vi "Continuous B-Scan Demo.vi"() -> ()   [LabVIEW 2012]
uses:
  LabVIEW/user.lib/SpectralRadar.llb/Device Camera Preset Selection.ctl
  LabVIEW/user.lib/SpectralRadar.llb/Raw Data Export Format Selection.ctl
  LabVIEW/user.lib/SpectralRadar.llb/set Spectrum Output.vi
  LabVIEW/user.lib/SpectralRadar.llb/set Scan Output.vi
  LabVIEW/user.lib/SpectralRadar.llb/display Data 2D.vi
  LabVIEW/user.lib/SpectralRadar.llb/OCT Device.lvclass
  LabVIEW/user.lib/SpectralRadar.llb/Probe.lvclass
  LabVIEW/user.lib/SpectralRadar.llb/Processing.lvclass
  LabVIEW/user.lib/SpectralRadar.llb/Raw Data.lvclass
  LabVIEW/user.lib/SpectralRadar.llb/Data.lvclass
  LabVIEW/user.lib/SpectralRadar.llb/Scan Pattern.lvclass
panel:
  in  "Raw Data Export Format":T1
  in  "Device Camera Preset":T2=enum."Preset 1"
  in  "Range":dbl=1.0
  in  "Path":path
  in  "stop":bool
  out "B-Scan Data":dbl[][](graph)
  out "Spectral Data":dbl[][](graph)
  in  "AScans":i32=512
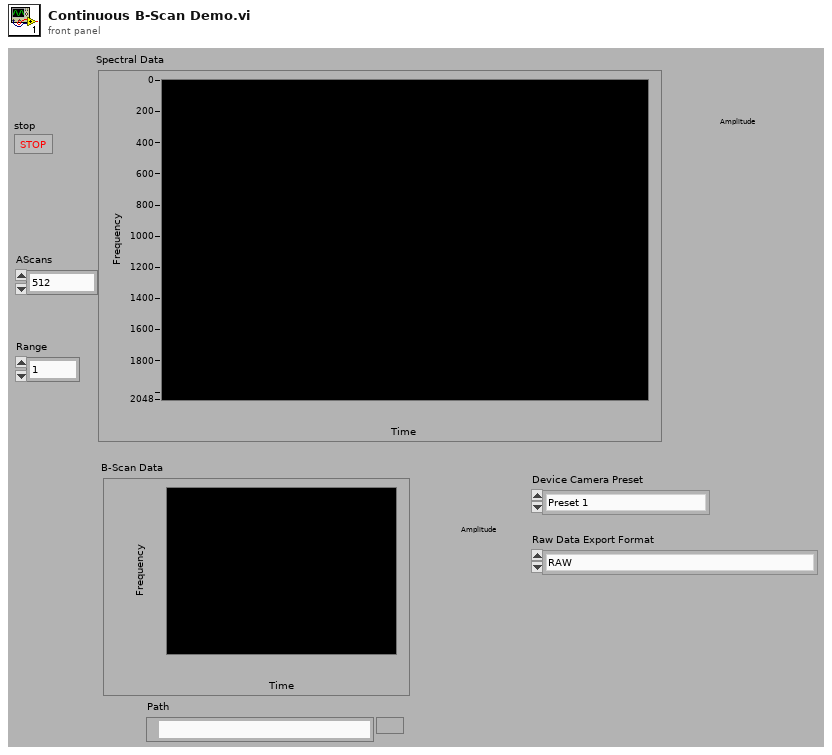
[diagram p1: front panel]
types:
  T1 = typedef "Raw Data.lvclass/Raw Data Export Format Selection.ctl" = enum16{"RAW", "SRR (Spectral Radar Raw)"}
  T2 = typedef "OCT Device.lvclass/Device Camera Preset Selection.ctl" = enum16{"Default", "Preset 1", "Preset 2", "Preset 3"}
  T3 = enum16{"Asynchronous Continuous", "Asynchronous Finite", "Synchronous"}
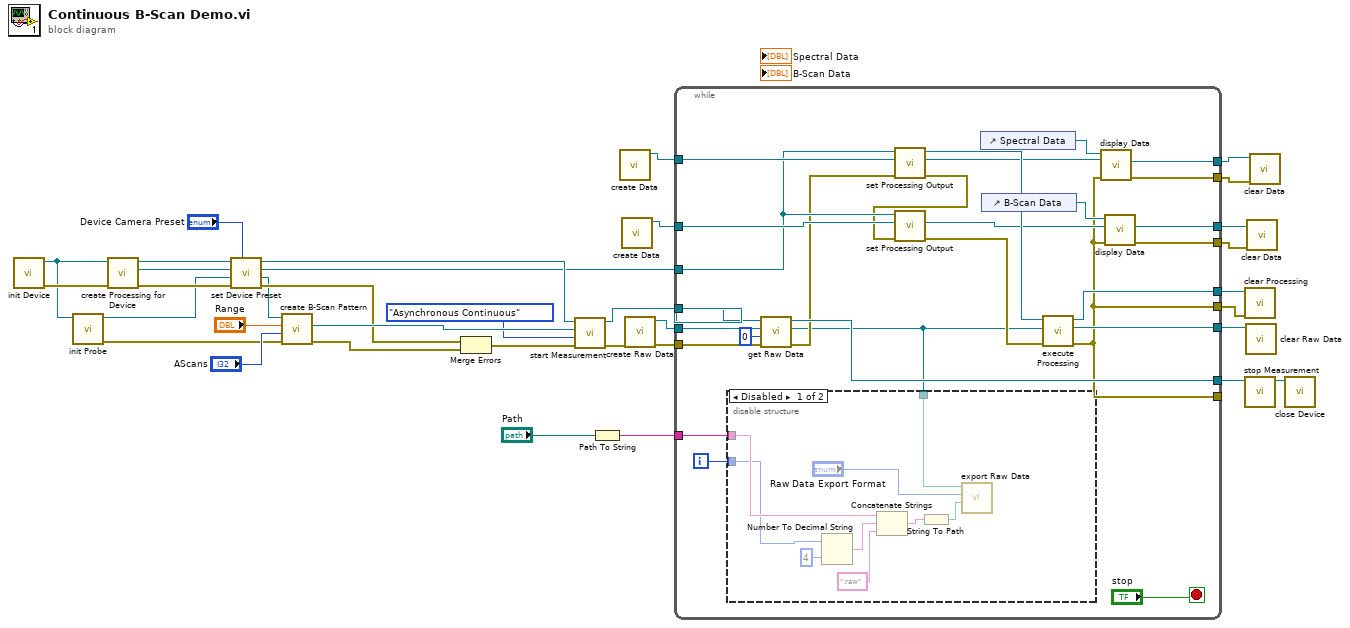
[diagram p0: block diagram]
diagram:
  n1 = call "init Device.vi"() -> ("error out"=w34:errorcluster, "OCTDevice"=w21:refnum<class "OCT Device.lvclass">)  [unwired: 6 in]
  n2 = call "init Probe.vi"("OCT Device"=w21) -> ("error out"=w20:errorcluster, "GalvoControl"=w15:refnum<class "Probe.lvclass">)  [unwired: 5 in]
  n3 = call "create Processing for Device.vi"("error in (no error)"=w34, "OCTDevice"=w21) -> ("error out"=w28:errorcluster, "Processing"=w13:refnum<class "Processing.lvclass">, "OCTDevice"=w16:refnum<class "OCT Device.lvclass">)  [unwired: 3 in]
  n4 = call "set Device Preset.vi"("Numeric"="Device Camera Preset", "Probe"=w15, "Processing"=w13, "OCTDevice"=w16) -> ("Probe 2"=w11:refnum<class "Probe.lvclass">, "Processing"=w12:refnum<class "Processing.lvclass">, "OCTDevice out"=w14:refnum<class "OCT Device.lvclass">)  [unwired: 2 in, 1 out]
  n5 = call "create B-Scan Pattern.vi"("error in (no error)"=w20, "AScans"="AScans", "Range"="Range", "Probe"=w11) -> ("error out"=w30:errorcluster, "Scan Pattern"=w32:refnum<class "Scan Pattern.lvclass">)  [unwired: 2 in, 1 out]
  n6 = Merge Errors(w28, w30) -> (w29:errorcluster)
  n7 = call "start Measurement.vi"("error in (no error)"=w29, "Acquisition Type"=T3."Asynchronous Continuous", "Scan Pattern"=w32, "OCTDevice"=w14) -> ("error out"=w26:errorcluster, "OCTDevice"=w17:refnum<class "OCT Device.lvclass">)  [unwired: 1 in, 1 out]
  n8 = Path To String(path="Path") -> (string=w9:string)
  n9 = call "create Data.vi"() -> ("Data"=w2:refnum<class "Data.lvclass">)  [unwired: 6 in, 1 out]
  n10 = call "create Data.vi"() -> ("Data"=w1:refnum<class "Data.lvclass">)  [unwired: 6 in, 1 out]
  n11 = call "create Raw Data.vi"("error in (no error)"=w26) -> ("error out"=w25:errorcluster, "Raw Data"=w27:refnum<class "Raw Data.lvclass">)  [unwired: 5 in]
  n12 = while {
    tunnel: w27 -> [w60]
    tunnel: w17 -> [w61]
    tunnel: w25 -> [w59]
    tunnel: w12 -> [w56]
    tunnel: w1 -> [w58]
    tunnel: w2 -> [w57]
    tunnel: [w48] -> w24
    tunnel: [w47] -> w23
    tunnel: [w46] -> w6
    tunnel: [w45] -> w4
    tunnel: [w44] -> w5
    tunnel: [w43] -> w3
    tunnel: [w42] -> w19
    tunnel: [w40] -> w22
    tunnel: [w40] -> _
    tunnel: w9 -> [w37]
    i -> [w36]
    stop <- "stop" stop-if-true
    n13 = call "get Raw Data.vi"("error in (no error)"=w59, "Camera Index"=0, "RawData in"=w60, "OCTDevice in"=w61) -> ("error out"=w41:errorcluster, "RawData out"=w38:refnum<class "Raw Data.lvclass">, "OCTDevice out"=w42:refnum<class "OCT Device.lvclass">)  [unwired: 1 in]
    n14 = disable-structure shown="Disabled" {
      disable-tunnel: w38 -> [w70 _]
      disable-tunnel: w37 -> [w69 _]
      disable-tunnel: w36 -> [w68 _]
      frame Disabled {
        n15 = Number To Decimal String(number=w68, width (-)=i16 4) -> (decimal integer string=w64:string)
        n16 = Concatenate Strings(w69, w64, ".raw" ("string")) -> (w65:string)
        n17 = String To Path(string=w65) -> (path=w66:path)
        n18 = call "export Raw Data.vi"("Export File"=w66, "Raw Data Export Format Selection"="Raw Data Export Format", "Data in"=w70) -> ()  [unwired: 3 in, 2 out]
      }
      frame Enabled {
      }
    }
    n19 = call-poly "set Processing Output.vi"("error in (no error)"=w41, "Data"=w57, "Processing"=w56) -> ("error out"=w54:errorcluster, "Data"=w51:refnum<class "Data.lvclass">, "Processing"=w55:refnum<class "Processing.lvclass">)  [unwired: 2 in]
    n20 = call-poly "set Processing Output.vi"("error in (no error)"=w54, "Data"=w58, "Processing"=w56) -> ("error out"=w53:errorcluster, "Data"=w49:refnum<class "Data.lvclass">)  [unwired: 2 in, 1 out]
    n21 = control-ref of="Spectral Data"() -> (w52:refnum<vi>)
    n22 = control-ref of="B-Scan Data"() -> (w50:refnum<vi>)
    n23 = call "execute Processing.vi"("error in (no error)"=w53, "Raw Data"=w38, "Processing"=w55) -> ("error out"=w40:errorcluster, "Raw Data"=w48:refnum<class "Raw Data.lvclass">, "Processing"=w47:refnum<class "Processing.lvclass">)  [unwired: 2 in]
    n24 = call-poly "display Data.vi"("error in (no error)"=w40, "Data in"=w51, "IntGraph Refnum"=w52) -> ("error out"=w43:errorcluster, "Data out"=w45:refnum<class "Data.lvclass">)  [unwired: 2 in, 1 out]
    n25 = call-poly "display Data.vi"("error in (no error)"=w40, "Data in"=w49, "IntGraph Refnum"=w50) -> ("error out"=w44:errorcluster, "Data out"=w46:refnum<class "Data.lvclass">)  [unwired: 2 in, 1 out]
  }
  n26 = call "clear Processing.vi"("error in (no error)"=w22, "Processing"=w23) -> ()  [unwired: 5 in, 1 out]
  n27 = call "stop Measurement.vi"("OCTDevice"=w19) -> ("OCTDevice"=w18:refnum<class "OCT Device.lvclass">)  [unwired: 5 in, 1 out]
  n28 = call "clear Raw Data.vi"("Raw Data"=w24) -> ()  [unwired: 6 in, 1 out]
  n29 = call "clear Data.vi"("error in (no error)"=w5, "Data"=w6) -> ()  [unwired: 5 in, 1 out]
  n30 = call "clear Data.vi"("error in (no error)"=w3, "Data"=w4) -> ()  [unwired: 5 in, 1 out]
  n31 = call "close Device.vi"("OCTDevice"=w18) -> ()  [unwired: 6 in, 1 out]
